vi "sutter_driver.vi"() -> ()   [LabVIEW 2016]
uses:
  <vilib>/Instr/_visa.llb/VISA Configure Serial Port (Instr).vi
panel:
  out "error out 2":errorcluster
  in  "y":cluster{"Go Home":bool, "Position":dbl[]}[](array[cluster])
  in  "Motor Poisition":dbl[][](array[numeric]) caption="Motor Poisition\nA               B"
  out "Position XYZ":dbl[](array[numeric])
  in  "Motor Select":u16(ring) items=["A"=1, "B"=2, "C"=3, "D"=4]
  in  "error in (no error)":errorcluster
  in  "stop":bool
  out "error out":errorcluster
  in  "VISA resource name":refnum<visa-resource-name>
  # "Motor Poisition\nA               B"
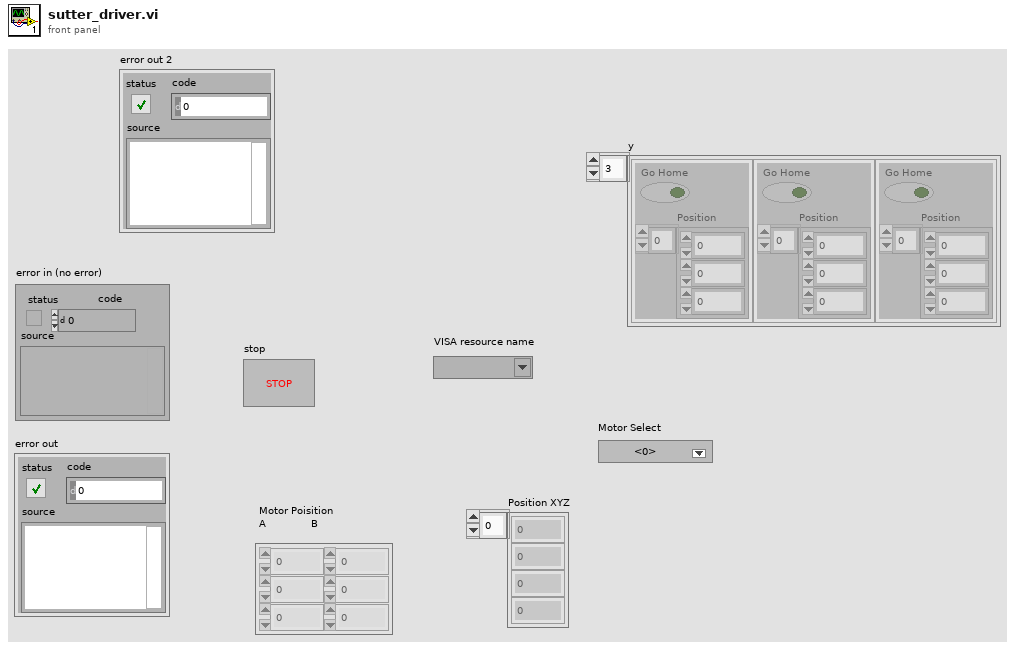
[diagram p1: front panel]
types:
  T1 = cluster{"Motor":u16, "Go Home":bool, "Position":dbl[]}
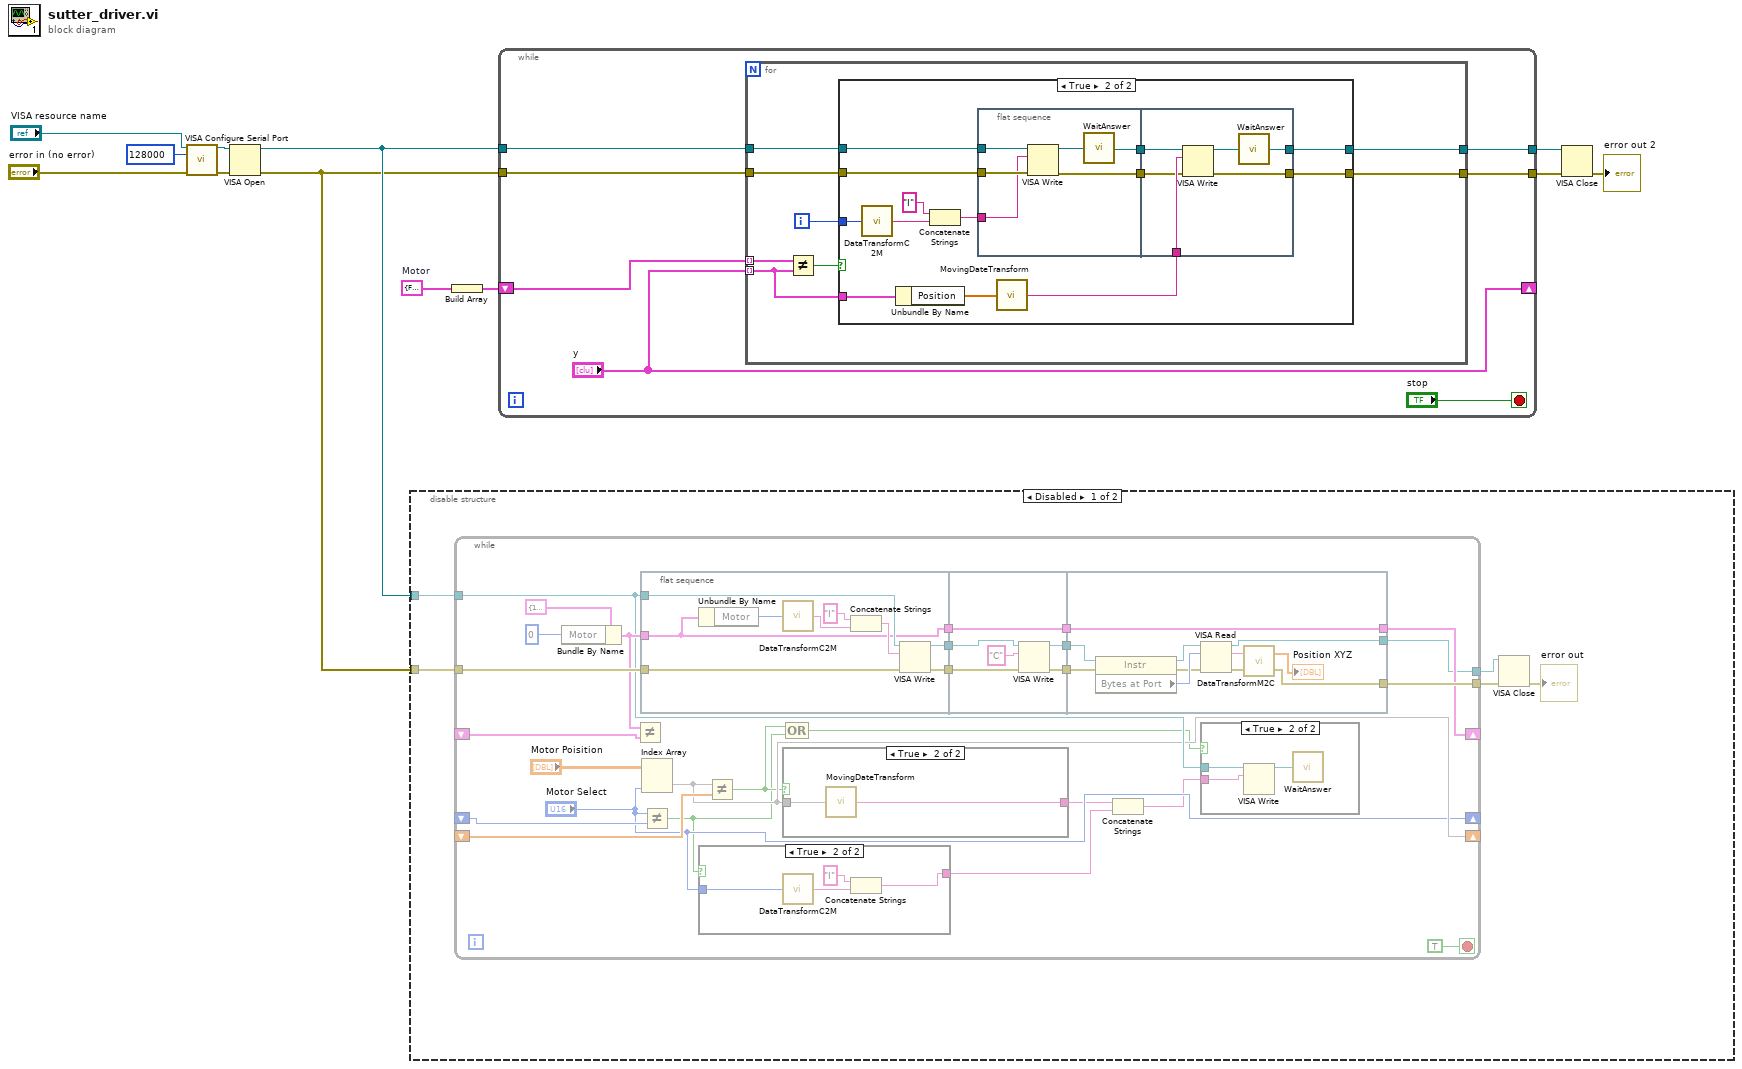
[diagram p0: block diagram]
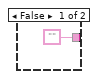
[diagram p2: hidden frame]
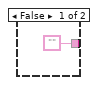
[diagram p3: hidden frame]
diagram:
  w5 = cluster{"Go Home":bool, "Position":dbl[]} {"Go Home"=FALSE, "Position"=[0.0, 0.0, 0.0]}  # Motor
  n1 = call-poly "VISA Configure Serial Port"("VISA resource name"="VISA resource name", "baud rate (9600)"=u32 128000, "error in (no error)"="error in (no error)") -> ("VISA resource name out"=w10:refnum<visa-resource-name>, "error out"=w8:errorcluster)  [unwired: 11 in]
  n2 = VISA Open(error in (no error)=w8, VISA resource name=w10) -> (VISA resource name=w7:refnum<visa-resource-name>, error out=w6:errorcluster)  [unwired: 3 in]
  n3 = disable-structure shown="Disabled" {
    disable-tunnel: w7 -> [w14 _]
    disable-tunnel: w6 -> [w13 _]
    frame Disabled {
      n4 = while {
        tunnel: w13 -> [w44]
        tunnel: [w37] -> w16
        tunnel: w14 -> [w38]
        tunnel: [w43] -> w15
        shift-right: [w41] -> _
        shift-left: _ -> [w42]
        shift-right: [w28] -> _
        shift-left: _ -> [w36]
        shift-right: ["Motor Select"] -> _
        shift-left: _ -> [w27]
        stop <- TRUE stop-if-true
        n5 = Bundle By Name(cluster=T1 {"Motor"=1, "Go Home"=FALSE, "Position"=[0.0, 0.0, 0.0]}, "Motor"=u16 0) -> (w39:T1)
        n6 = Not Equal?(x=w39, y=w42) -> ()  [unwired: 1 out]
        n7 = flat-sequence {
          tunnel: w44 -> [w58]
          tunnel: w38 -> [w61]
          tunnel: w39 -> [w53]
          tunnel: [w55] -> w32
          tunnel: [w54] -> w31
          tunnel: [w53] -> w30
          tunnel: [w66] -> w35
          tunnel: [w65] -> w34
          tunnel: [w62] -> w33
          tunnel: w32 -> [w64]
          tunnel: w31 -> [w63]
          tunnel: w30 -> [w62]
          tunnel: w35 -> [w76]
          tunnel: [w75] -> w37
          tunnel: w34 -> [w74]
          tunnel: w33 -> [w72]
          tunnel: [w72] -> w41
          tunnel: [w68] -> w43
          frame #0 {
            n8 = Unbundle By Name(w53) -> ("Motor"=w57:u16)
            n9 = call "DataTransformC2M.vi"("input"=w57) -> ("output"=w56:string)
            n10 = Concatenate Strings("I" ("string"), w56) -> (w60:string)
            n11 = VISA Write(VISA resource name=w61, write buffer=w60, error in (no error)=w58) -> (VISA resource name out=w55:refnum<visa-resource-name>, error out=w54:errorcluster)  [unwired: 1 out]
          }
          frame #1 {
            n12 = VISA Write(VISA resource name=w64, write buffer="C", error in (no error)=w63) -> (VISA resource name out=w66:refnum<visa-resource-name>, error out=w65:errorcluster)  [unwired: 1 out]
          }
          frame #2 {
            n13 = property class="Instr"(reference=w76, error in=w74) -> (reference out=w78:refnum<visa-resource-name>, error out=w73:errorcluster, "Bytes at Port"=w77:u32)
            n14 = VISA Read(VISA resource name=w78, byte count=w77, error in (no error)=w73) -> (VISA resource name out=w75:refnum<visa-resource-name>, read buffer=w71:string, error out=w70:errorcluster)  [unwired: 1 out]
            n15 = call "DataTransformM2C.vi"("ERROR IN"=w70, "MotorData"=w71) -> ("ERROR OUT"=w68:errorcluster, "Computer Data"=→"Position XYZ":dbl[])
          }
        }
        n16 = Index Array(array="Motor Poisition", index (col)="Motor Select") -> (element=w28:dbl[])  [unwired: 1 in]
        n17 = Not Equal?(x="Motor Select", y=w27) -> (x != y?=w19:bool)
        n18 = case shown="True" w19 {
          tunnel: "Motor Select" -> [_ w47]
          tunnel: ["" w46] -> w23
          frame False {
          }
          frame True {
            n19 = call "DataTransformC2M.vi"("input"=w47) -> ("output"=w48:string)
            n20 = Concatenate Strings("I" ("string"), w48) -> (w46:string)
          }
        }
        n21 = Not Equal?(x=w28, y=w36) -> (x != y?=w21:bool)
        n22 = case shown="True" w21 {
          tunnel: w28 -> [_ w52]
          tunnel: ["" w51] -> w24
          frame False {
          }
          frame True {
            n23 = call "MovingDateTransform.vi"("INPUT"=w52) -> ("MOVEING COMMAND"=w51:string)  [unwired: 2 in]
          }
        }
        n24 = Compound Arithmetic op=OR ("复合运算")(w21, w19) -> (w20:bool)
        n25 = Concatenate Strings(w24, w23) -> (w22:string)
        n26 = case shown="True" w20 {
          tunnel: w38 -> [_ w81]
          tunnel: w22 -> [_ w80]
          frame False {
          }
          frame True {
            n27 = VISA Write(VISA resource name=w81, write buffer=w80) -> (VISA resource name out=w79:refnum<visa-resource-name>)  [unwired: 1 in, 2 out]
            n28 = call "WaitAnswer.vi"("VISA resource name in"=w79) -> ()  [unwired: 1 out]
          }
        }
      }
      n29 = VISA Close(VISA resource name=w16, error in (no error)=w15) -> (error out=→"error out":errorcluster)
    }
    frame Enabled {
    }
  }
  n30 = Build Array(w5) -> (w4:cluster{"Go Home":bool, "Position":dbl[]}[])
  n31 = while {
    tunnel: w7 -> [w87]
    tunnel: w6 -> [w86]
    shift-right: ["y"] -> _
    shift-left: w4 -> [w88]
    tunnel: [w83] -> w2
    tunnel: [w82] -> w1
    stop <- "stop" stop-if-true
    n32 = for {
      tunnel: w88 -> [w96] mode=indexing
      tunnel: "y" -> [w91] mode=indexing
      tunnel: w87 -> [w94]
      tunnel: w86 -> [w92]
      tunnel: [w90] -> w83
      tunnel: [w89] -> w82
      i -> [w93]
      n33 = Not Equal?(x=w96, y=w91) -> (x != y?=w95:bool)
      n34 = case shown="True" w95 {
        tunnel: w94 -> [w98 w111]
        tunnel: w93 -> [_ w102]
        tunnel: w92 -> [w97 w110]
        tunnel: w91 -> [_ w109]
        tunnel: [w98 w100] -> w90
        tunnel: [w97 w99] -> w89
        frame False {
        }
        frame True {
          n35 = call "DataTransformC2M.vi"("input"=w102) -> ("output"=w103:string)
          n36 = Unbundle By Name(w109) -> ("Position"=w108:dbl[])
          n37 = Concatenate Strings("I" ("string"), w103) -> (w101:string)
          n38 = flat-sequence {
            tunnel: w111 -> [w117]
            tunnel: w110 -> [w116]
            tunnel: [w114] -> w107
            tunnel: [w113] -> w105
            tunnel: w101 -> [w112]
            tunnel: w107 -> [w122]
            tunnel: w106 -> [w121]
            tunnel: w105 -> [w120]
            tunnel: [w119] -> w100
            tunnel: [w118] -> w99
            frame #0 {
              n39 = VISA Write(VISA resource name=w117, write buffer=w112, error in (no error)=w116) -> (VISA resource name out=w115:refnum<visa-resource-name>, error out=w113:errorcluster)  [unwired: 1 out]
              n40 = call "WaitAnswer.vi"("VISA resource name in"=w115) -> ("VISA resource name out"=w114:refnum<visa-resource-name>)
            }
            frame #1 {
              n41 = VISA Write(VISA resource name=w122, write buffer=w121, error in (no error)=w120) -> (VISA resource name out=w123:refnum<visa-resource-name>, error out=w118:errorcluster)  [unwired: 1 out]
              n42 = call "WaitAnswer.vi"("VISA resource name in"=w123) -> ("VISA resource name out"=w119:refnum<visa-resource-name>)
            }
          }
          n43 = call "MovingDateTransform.vi"("INPUT"=w108) -> ("MOVEING COMMAND"=w106:string)  [unwired: 2 in]
        }
      }
    }
  }
  n44 = VISA Close(VISA resource name=w2, error in (no error)=w1) -> (error out=→"error out 2":errorcluster)
